vi "OCV FPS.vi"() -> (3 "FPS":dbl, 4 "Last Frame Time, ms":u32)   [LabVIEW 2018, in "OpenCVcamLV.lvlib"]
doc: "Calculate the frame rate from within a loop. Frame rate is averaged over the specified update interval. The default update interval is 1000ms."
uses:
  OpenCVcamLV.lvlib
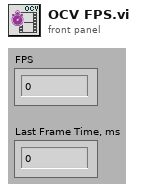
[diagram p1: front panel]
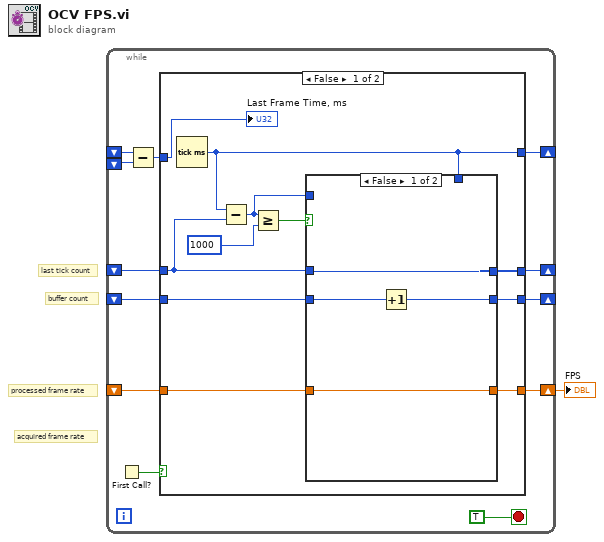
[diagram p0: block diagram]
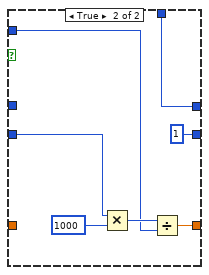
[diagram p2: hidden frame]
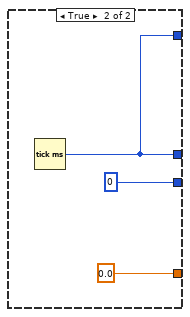
[diagram p3: hidden frame]
diagram:
  # "processed frame rate"
  # "buffer count"
  # "acquired frame rate"
  # "last tick count"
  n1 = while {
    shift-right: [w11] -> _
    shift-left: _ -> [w10]
    shift-right: [w9] -> _
    shift-left: _ -> [w8]
    shift-right: [w7] -> w1
    shift-left: _ -> [w6]
    shift-right: [w5] -> _
    shift-left: _ -> [w4]
    shift-left: _ -> [w3]
    stop <- TRUE stop-if-true
    n2 = First Call?() -> (First Call?: T/F=w12:bool)
    n3 = Subtract(x=w4, y=w3) -> (x-y=w2:u32)
    n4 = case shown="False" w12 {
      tunnel: [w21 w37] -> w11
      tunnel: w10 -> [w22 _]
      tunnel: [w18 u32 0 ("buffer number")] -> w9
      tunnel: w8 -> [w19 _]
      tunnel: [w17 0.0] -> w7
      tunnel: w6 -> [w16 _]
      tunnel: [w15 w37] -> w5
      tunnel: w2 -> [w14 _]
      frame False {
        n5 = Tick Count (ms)() -> (millisecond timer value=w15:u32)
        n6 = Subtract(x=w15, y=w22) -> (x-y=w20:u32)
        n7 = Greater Or Equal?(x=w20, y=u32 1000 ("Update interval")) -> (x >= y?=w23:bool)
        n8 = case shown="False" w23 {
          tunnel: w22 -> [w28 _]
          tunnel: [w28 w35] -> w21
          tunnel: w15 -> [_ w35]
          tunnel: w20 -> [_ w30]
          tunnel: w19 -> [w27 w32]
          tunnel: [w26 u32 1] -> w18
          tunnel: [w25 w29] -> w17
          tunnel: w16 -> [w25 _]
          frame False {
            n9 = Increment(x=w27) -> (x+1=w26:u32)
          }
          frame True {
            n10 = Multiply(x=w32, y=u32 1000) -> (x*y=w31:u32)
            n11 = Divide(x=w31, y=w30) -> (x/y=w29:dbl)
          }
        }
        "Last Frame Time, ms" <- w14
      }
      frame True {
        n12 = Tick Count (ms)() -> (millisecond timer value=w37:u32)
      }
    }
  }
  "FPS" <- w1
